vi "Robot Global Data(2).vi"() -> ()   [LabVIEW 2013]
doc: "This global VI can contain as many global variables as you need. Place a control on the panel, give it a good name. To read or write to it from a VI, drag the icon to the diagram of that VI. You can also drag from the project. Click on the node to change which global you access. You shouldn't have multiple locations writing to a global or it will cause a race-condition."
uses:
  <vilib>/Rock Robotics/WPI/Camera/WPI_CameraImageSize.ctl
  <vilib>/Rock Robotics/WPI/DriverStation/WPI_DriverStationRobotMode2.ctl
panel:
  in  "Starting time 2":dbl
  in  "Gear Box Servo Value":dbl=-1.0
  in  "Defender State":dbl
  in  "Defender value":dbl=-1.0
  in  "Defender":bool
  in  "Waiting For Event":string
  in  "Aux Button Pressed":bool
  in  "Simulation Mode":bool
  in  "Gearbox Limit B":bool
  in  "Gearbox Limit F":bool
  in  "Fire Limit B":bool
  in  "Fire Limit F":bool
  in  "Arm Limit B":bool
  in  "Arm Limit F":bool
  in  "Gear Box button":bool
  in  "Gear Box Value":dbl=-1.0
  in  "Current State Name":string
  in  "Starting time":dbl
  in  "Test":dbl
  in  "Vacuum Button":bool
  in  "VacuumLatched button":dbl=-1.0
  in  "State Machine":T1(ring)
  in  "Robot Mode":T2
  in  "LED toggle rate (ms)":u32=20
  in  "image size":T3=enum."320x240"
  in  "Enable Vision":bool
  # "Our Global Variables"
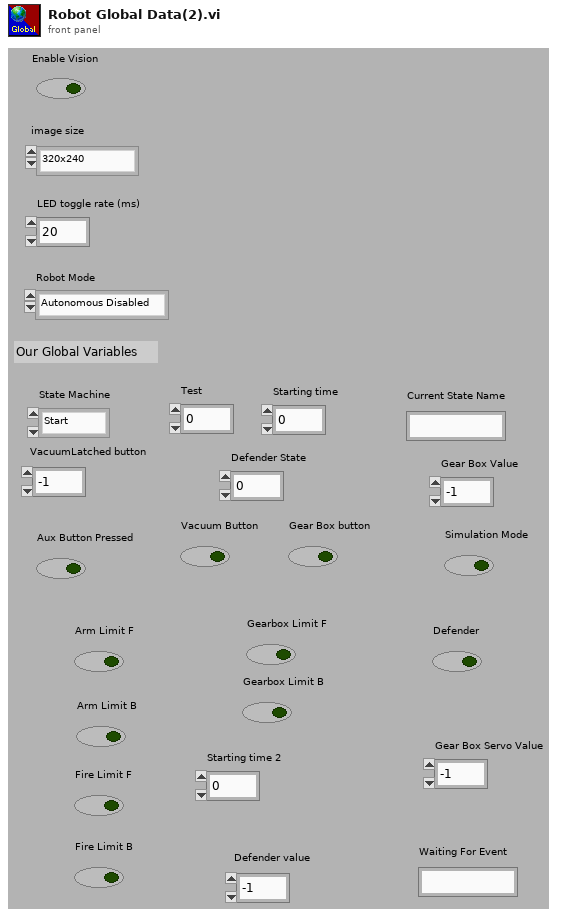
[diagram p1: front panel]
types:
  T1 = enum16{"Start", "Reset", "Reset 2", "Reset Delay", "Reset 3", "Manual", "Wait for Firing Latch", "Get ready to Fire", "Disengage Gearbox", "Ready to Fire", "Firing", "Firing Completed", "Reengage Gearbox"}
  T2 = typedef "WPI_DriverStationRobotMode2.ctl" = enum16{"Autonomous Disabled", "Autonomous Enabled", "Teleop Disabled", "Teleop Enabled", "Timeout", "Finish", "Test Disabled", "Test Enabled"}
  T3 = typedef "WPI_CameraImageSize.ctl" = enum16{"640x480", "320x240", "160x120"}
diagram:
